vi "RSZVB Set Frequency Conversion.vi"(0 "VISA session":refnum<visa-resource-name>, 1 "Denominator (1)":i32=1, 2 "Sweep Type (0: Sweep)":i32(ring) items=["Sweep", "CW/Fixed"], 5 "Measurement Type (0: Receiver)":i32(ring) items=["Receiver", "Source"], 7 "Channel (1)":i32=1, 9 "Port (1)":i32=1, 11 "error in (no error)":errorcluster {"code" format="%.0x"}, 12 "Offset (0.0)":dbl format="%^.3e", 13 "Numerator (1)":i32=1) -> (4 "dup VISA session":refnum<visa-resource-name>, 15 "error out":errorcluster {"code" format="%.0x"})   [LabVIEW 2011]
doc: "This VI defines the receiver frequency or the port-specific source frequency for frequency-converting measurements. The receiver/source frequency is either a range (for frequency sweeps) or a CW frequency (for power, time and CW Mode sweeps). The receiver frequency is valid for all ports. \n\nRemote-control command(s):\n[SENSe<Ch>:]FREQuency:CONVersion:ARBitrary <numerator>, <denominator>, <offset>, CW | FIXed | SWEep\nSOURce<Ch>:FREQuency<Pt>:CONVersion:ARBitrary:IFRequency <numerator>, <denominator>, <offset>, CW | FIXed | SWEep"
uses:
  _utility/RSZVB Global Data.vi
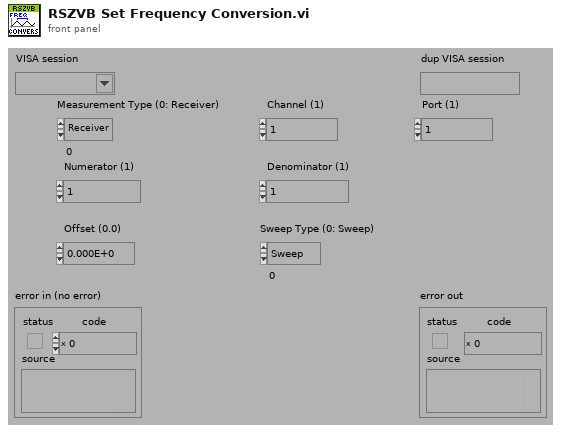
[diagram p1: front panel]
types:
  T1 = cluster{"Error Checking (T: On)":bool, "Installed Options":string[], "Data Valid?":bool, "Ports":i32, "Model":string[], "Option Checking (T: On)":bool}[]
  T2 = cluster{"Error Checking (T: On)":bool, "Installed Options":string[], "Data Valid?":bool, "Ports":i32, "Model":string[], "Option Checking (T: On)":bool}
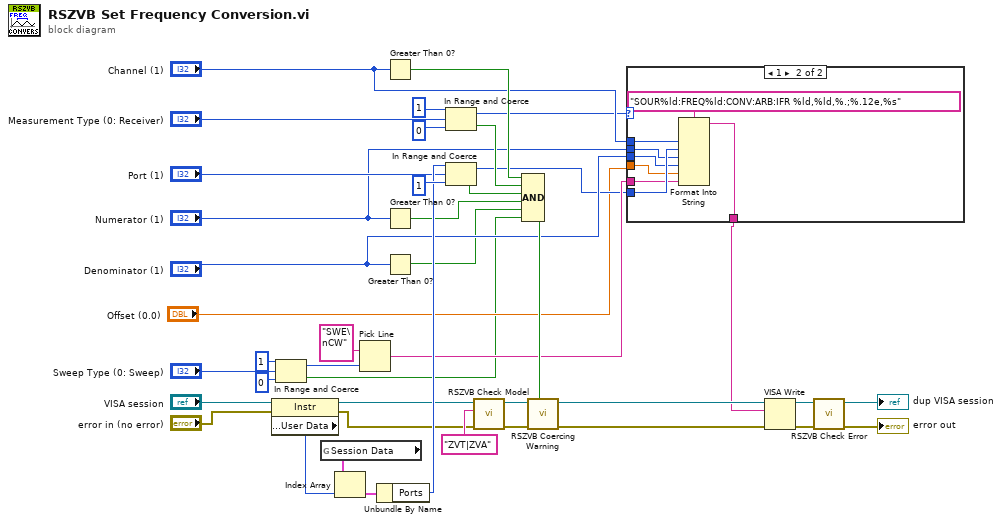
[diagram p0: block diagram]
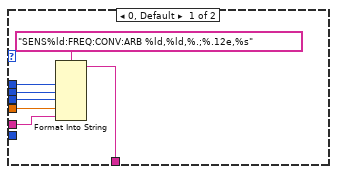
[diagram p2: hidden frame]
diagram:
  n1 = property class="Instr"(reference="VISA session", error in="error in (no error)") -> (reference out=w4:refnum<visa-resource-name>, error out=w3:errorcluster, "General Settings:User Data"=w39:u32)
  n2 = In Range and Coerce(upper limit=1 ("lower limit"), x="Sweep Type (0: Sweep)", lower limit=0) -> (coerced(x)=w18:i32, In Range?=w1:bool)
  n3 = global read "RSZVB Global Data.vi" "Session Data"() -> (w38:T1)
  n4 = Index Array(array=w38, index=w39) -> (element=w37:T2)
  n5 = Pick Line(multi-line string="SWE\nCW", line index=w18) -> (output string=w14:string)  [unwired: 1 in]
  n6 = Unbundle By Name(w37) -> ("Ports"=w26:i32)
  n7 = Greater Than 0?(x="Channel (1)") -> (x > 0?=w36:bool)
  n8 = Greater Than 0?(x="Numerator (1)") -> (x > 0?=w11:bool)
  n9 = Greater Than 0?(x="Denominator (1)") -> (x > 0?=w10:bool)
  n10 = In Range and Coerce(upper limit=1 ("lower limit"), x="Measurement Type (0: Receiver)", lower limit=0) -> (coerced(x)=w17:i32, In Range?=w42:bool)
  n11 = In Range and Coerce(upper limit=w26, x="Port (1)", lower limit=1) -> (coerced(x)=w13:i32, In Range?=w12:bool)
  n12 = call "RSZVB Check Model.vi"("error in (no error)"=w3, "Model"="ZVT|ZVA" ("Options"), "VISA session"=w4) -> ("error out"=w6:errorcluster, "dup VISA session"=w5:refnum<visa-resource-name>)  [unwired: 7 in]
  n13 = Compound Arithmetic op=AND(w36, w42, w12, w11, w10, w1) -> (w35:bool)
  n14 = call "RSZVB Coercing Warning.vi"("In Range?"=w35, "error in (no error)"=w6, "VISA session"=w5) -> ("error out"=w9:errorcluster, "dup VISA session"=w32:refnum<visa-resource-name>)  [unwired: 7 in]
  n15 = case shown="1" w17 {
    tunnel: "Numerator (1)" -> [w49 w54]
    tunnel: "Offset (0.0)" -> [w48 w52]
    tunnel: [w47 w50] -> w8
    tunnel: "Channel (1)" -> [w45 w56]
    tunnel: "Denominator (1)" -> [w44 w53]
    tunnel: w14 -> [w43 w51]
    tunnel: w13 -> [_ w55]
    frame 0, Default {
      n16 = Format Into String(format string="SENS%ld:FREQ:CONV:ARB %ld,%ld,%.;%.12e,%s", w45, w49, w44, w48, w43) -> (resulting string=w47:string)  [unwired: 2 in, 1 out]
    }
    frame 1 {
      n17 = Format Into String(format string="SOUR%ld:FREQ%ld:CONV:ARB:IFR %ld,%ld,%.;%.12e,%s", w56, w55, w54, w53, w52, w51) -> (resulting string=w50:string)  [unwired: 2 in, 1 out]
    }
  }
  n18 = VISA Write(VISA resource name=w32, write buffer=w8, error in (no error)=w9) -> (VISA resource name out=w34:refnum<visa-resource-name>, error out=w33:errorcluster)  [unwired: 1 out]
  n19 = call "RSZVB Check Error.vi"("error in (no error)"=w33, "VISA session"=w34) -> ("error out"=→"error out":errorcluster, "dup VISA session"=→"dup VISA session":refnum<visa-resource-name>)  [unwired: 8 in]
